vi "Check Status.vi"(8 "error in (no error)":errorcluster, 11 "Keithley Multimeter in":refnum<class "Testing Keithley Multimeter.lvclass">) -> (0 "error out":errorcluster, 1 "Status":string, 2 "Ready?":bool, 3 "Keithley Multimeter out":refnum<class "Testing Keithley Multimeter.lvclass">)   [LabVIEW 2017, in "Testing Keithley Multimeter.lvclass"]
doc: "(Dynamic) Check if the instrument is powered on and update its member fields with the instrument's current status. Optionally return a text status message."
uses:
  Testing Keithley Multimeter.lvclass
  Testing Keithley Multimeter.lvclass/Testing Keithley Multimeter.ctl
  Utility Classes/Readable/Readable.lvclass
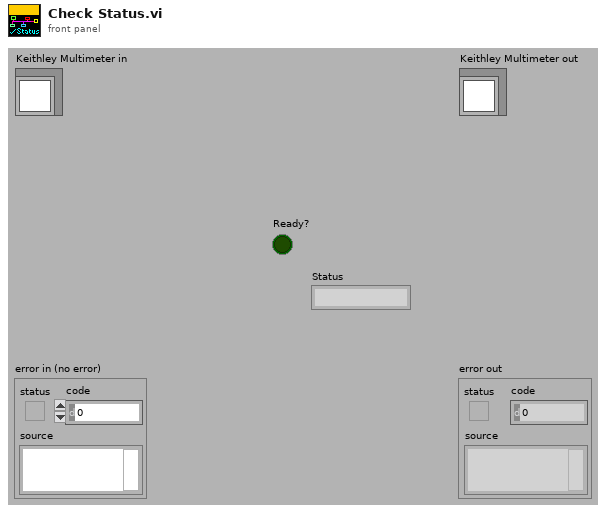
[diagram p1: front panel]
types:
  T1 = cluster{"error":bool, "code":i32, "source":string}
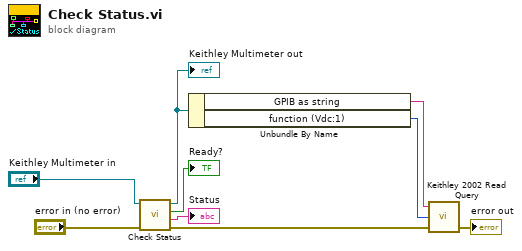
[diagram p0: block diagram]
diagram:
  n1 = call-parent "Check Status.vi"("error in (no error)"="error in (no error)", "Instrument in"="Keithley Multimeter in") -> ("error out"=w5:errorcluster, "Status"=→"Status":string, "Ready?"=→"Ready?":bool, "Instrument out"=w3:refnum<class "Testing Keithley Multimeter.lvclass">)  [unwired: 6 in]
  "Keithley Multimeter out" <- w3
  n2 = Unbundle By Name(w3) -> ("GPIB as string"=w2:string, "function (Vdc:1)"=w1:u16)
  n3 = call "Keithley 2002 Read Query.vi"("error in"=w5, "function (Vdc:1)"=w1, "GPIB Address"=w2) -> ("error out"=→"error out":T1)  [unwired: 1 in, 1 out]
